vi "Set Average.vi"(8 "error in (no error)":errorcluster, 9 "Average Factor":i32, 10 "Average?":enum16{"ON", "OFF"}(ring), 11 "Instrument.VSource in":refnum<class "VNA.lvclass">) -> (0 "error out":errorcluster, 3 "Instrument.VSource out":refnum<class "VNA.lvclass">)   [LabVIEW 2016, in "VNA.lvclass"]
uses:
  VNA.lvclass
  VNA.lvclass/VNA.ctl
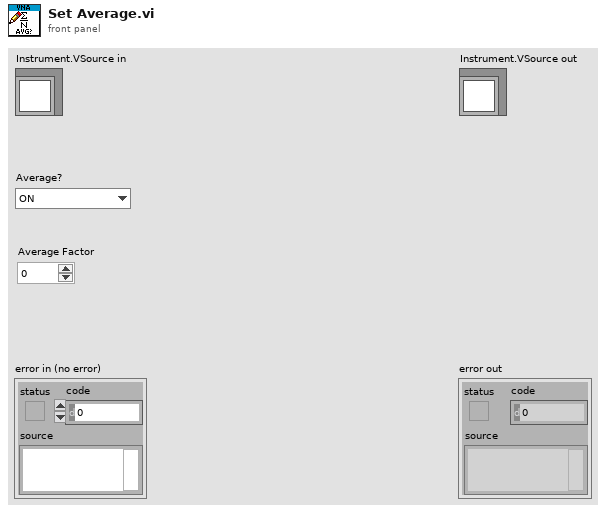
[diagram p1: front panel]
types:
  T1 = cluster{"Average?":enum16{"ON", "OFF"}, "Average Factor":i32}
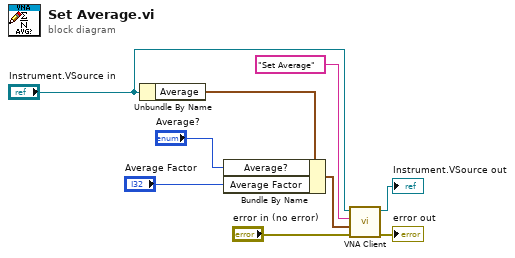
[diagram p0: block diagram]
diagram:
  n1 = Unbundle By Name("Instrument.VSource in") -> ("Average"=w1:T1)
  n2 = Bundle By Name(cluster=w1, "Average?"="Average?", "Average Factor"="Average Factor") -> (w3:T1)
  n3 = call "VNA Client.vi"("error in (no error)"="error in (no error)", "Data"=w3, "Command"="Set Average", "VNA in"="Instrument.VSource in") -> ("error out"=→"error out":errorcluster, "VNA out"=→"Instrument.VSource out":refnum<class "VNA.lvclass">)  [unwired: 6 in]
